vi "XLP80_CAN_PeakToNI.vi"(8 "error in":errorcluster, 11 "PEAK CANData Read":T1[](array[typedef]) {"ID" format="%.0x"}) -> (0 "error out":errorcluster, 3 "NI Data OUT":variant)   [LabVIEW 2021]
uses:
  <userlib>/PCAN Basic/Controls/CAN MSG Cluster.ctl
  <vilib>/nican/nican.llb/CanFrameTimed.ctl
  <userlib>/PCAN Basic/PCANBasic.lvlib
panel:
  out "DATA":u8[](array[numeric])
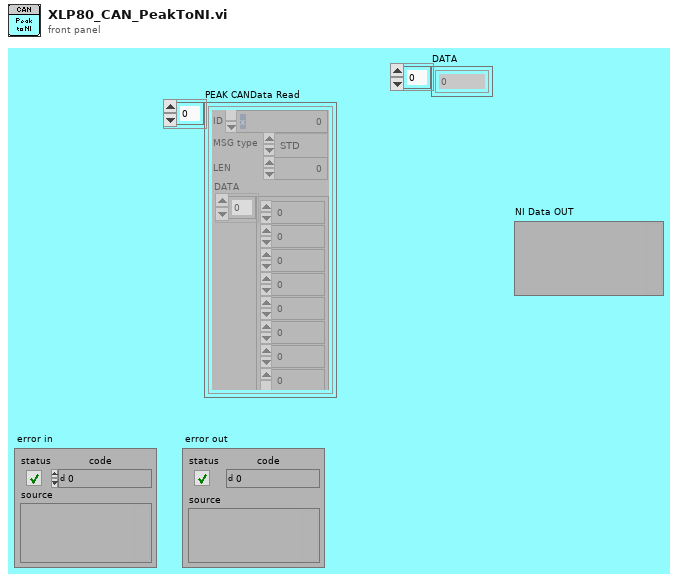
[diagram p1: front panel]
types:
  T1 = typedef "PCANBasic.lvlib/CAN MSG Cluster.ctl" = cluster{"ID":u32, "MSG type":enum8{"STD", "RTR", "XTD", "XTD RTR", "STATUS"}, "LEN":i8, "DATA":u8[]}
  T2 = typedef "CanFrameTimed.ctl" = cluster{"Timestamp":dbl, "ArbitrationId":u32, "IsRemote":u8, "DataLength":u8, "Data":u8[]}
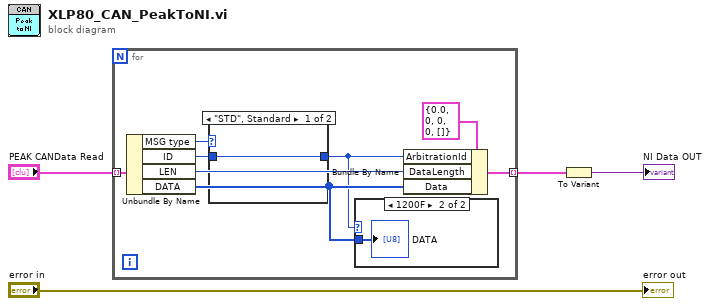
[diagram p0: block diagram]
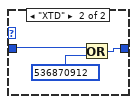
[diagram p2: hidden frame]
diagram:
  n1 = for {
    tunnel: "PEAK CANData Read" -> [w11] mode=indexing
    tunnel: [w9] -> w2 mode=indexing
    n2 = Unbundle By Name(w11) -> ("MSG type"=w7:enum8{"STD", "RTR", "XTD", "XTD RTR", "STATUS"}, "ID"=w6:u32, "LEN"=w10:i8, "DATA"=w8:u8[])
    n3 = case shown="\"STD\", Standard" w7 {
      tunnel: w6 -> [w13 w15]
      tunnel: [w13 w14] -> w5
      frame "STD", Default {
      }
      frame "XTD" {
        n4 = Or(x=w15, y=u32 536870912) -> (x .or. y?=w14:u32)
      }
    }
    n5 = case shown="1200F" w5 {
      tunnel: w8 -> [_ w17]
      frame 0, Default {
      }
      frame 73743 {
        "DATA" <- w17
      }
    }
    n6 = Bundle By Name(cluster=T2 {"Timestamp"=0.0, "ArbitrationId"=0, "IsRemote"=0, "DataLength"=0, "Data"=[]} ("CAN FRAME TIMED"), "ArbitrationId"=w5, "DataLength"=w10, "Data"=w8) -> (w9:T2)
  }
  n7 = To Variant(anything=w2) -> (Variant=→"NI Data OUT":variant)
  "error out" <- "error in"
